vi "EEPROM.vi"(11 "Address":u16 format="%04x") -> (3 "Data":u8 format="%.0x")   [LabVIEW 2021]
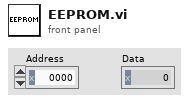
[diagram p1: front panel]
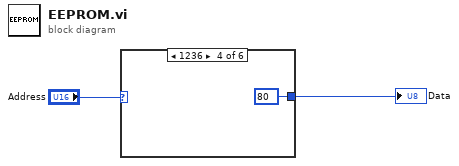
[diagram p0: block diagram]
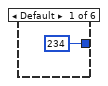
[diagram p2: hidden frame]
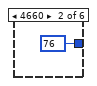
[diagram p3: hidden frame]
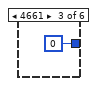
[diagram p4: hidden frame]
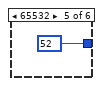
[diagram p5: hidden frame]
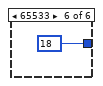
[diagram p6: hidden frame]
diagram:
  n1 = case shown="1236" "Address" {
    tunnel: [u8 234 u8 76 u8 0 u8 80 u8 52 u8 18] -> w2
    frame Default {
    }
    frame 4660 {
    }
    frame 4661 {
    }
    frame 4662 {
    }
    frame 65532 {
    }
    frame 65533 {
    }
  }
  "Data" <- w2
